vi "CRYPEAQ SpreadCB Sub.vi"(9 "Bs":dbl[](array[numeric]), 10 "Center Frequency":dbl[](array[numeric]), 11 "E":dbl[](array[numeric])) -> (3 "Es":dbl[](array[numeric]))   [LabVIEW 2013]
panel:
  out "Array 2":dbl[](array[numeric])
  out "Array":dbl[](array[numeric])
  out "aUCEe":dbl[](array[numeric])
  out "Ene":dbl[](array[numeric])
  in  "res":dbl=0.25
  out "XY Graph 4":cluster{"Center Frequency":dbl[], "E":dbl[]}[](graph)
  out "size(s) 4":i32
  out "size(s) 3":i32
  out "size(s)":i32
  # "SU Value Range"
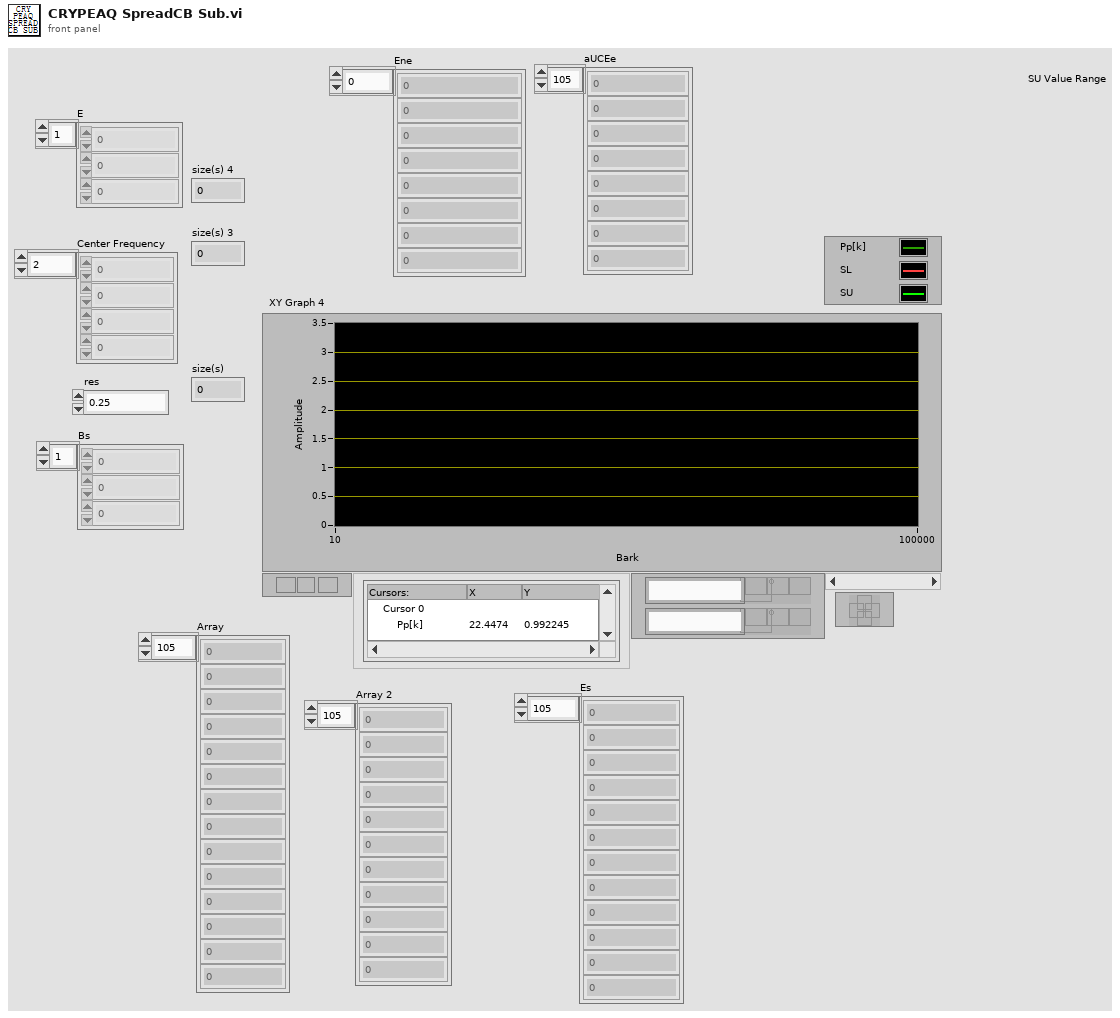
[diagram p1: front panel]
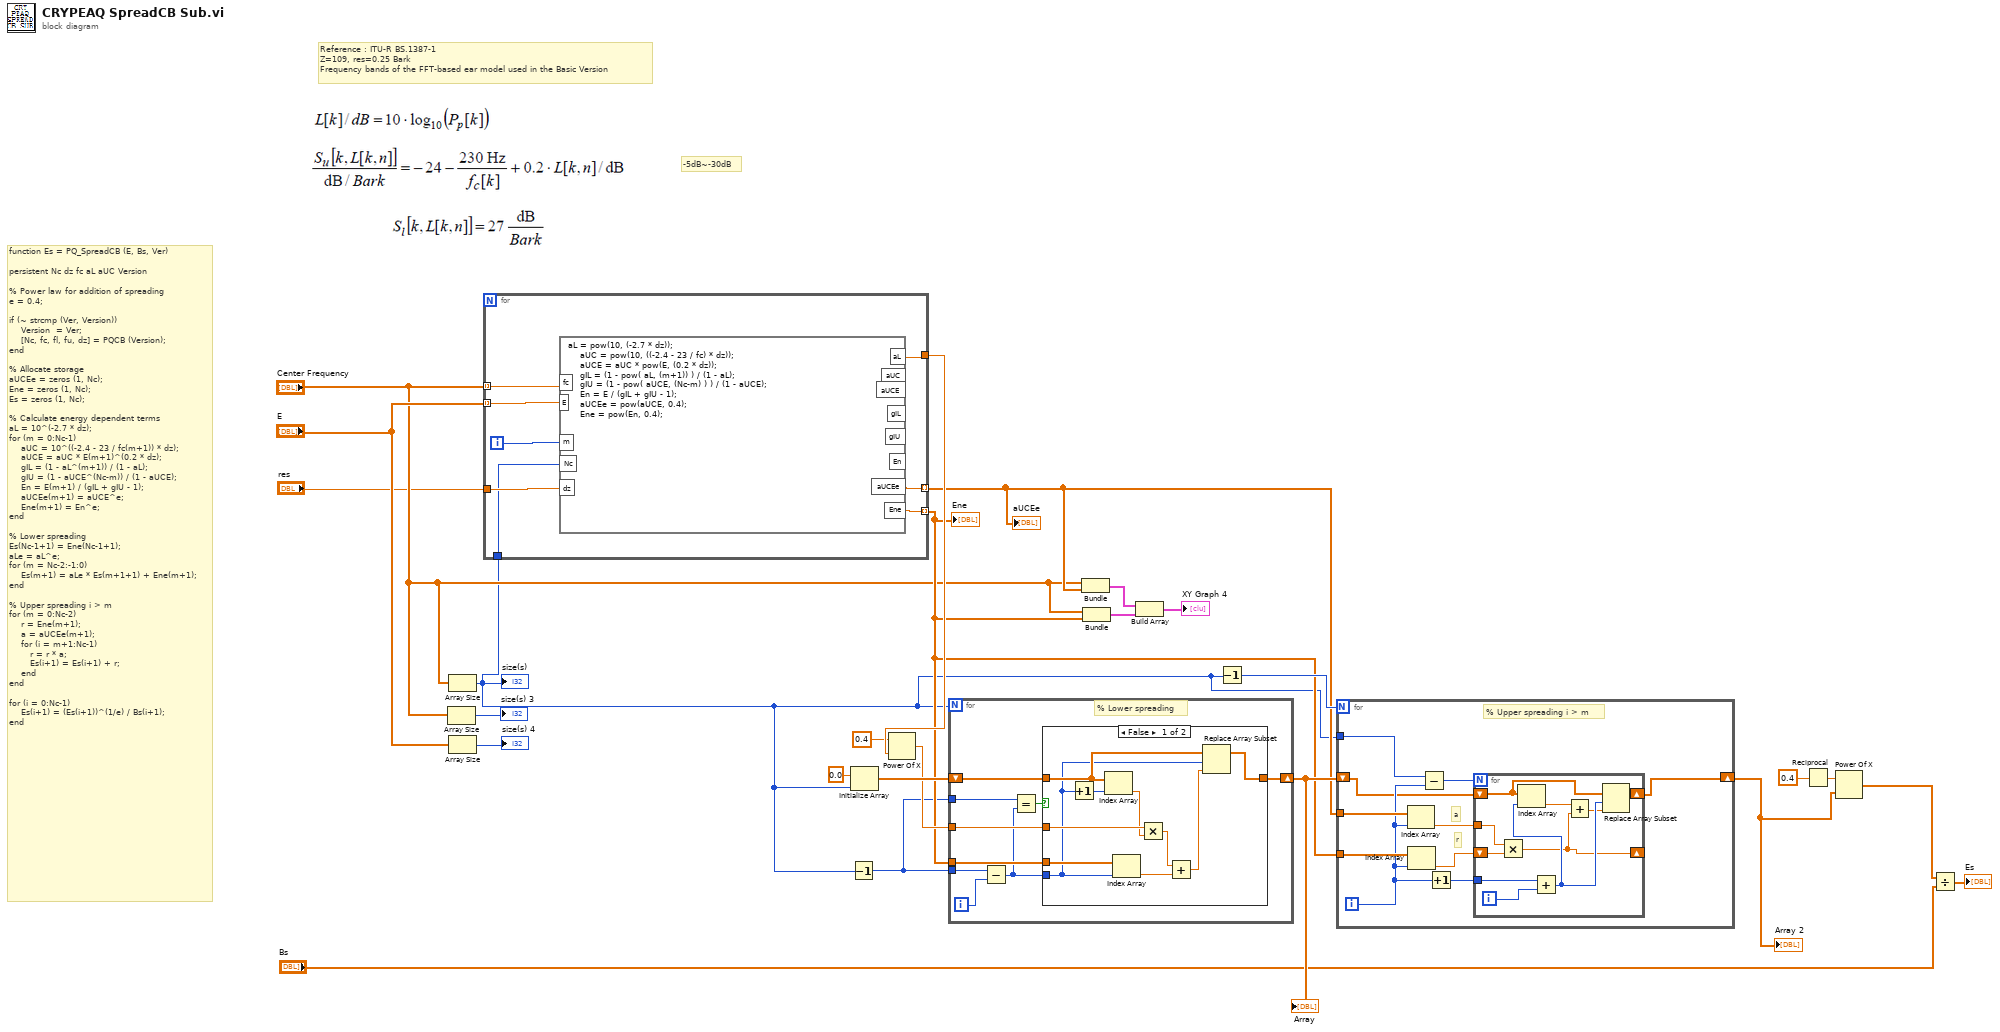
[diagram p0: block diagram]
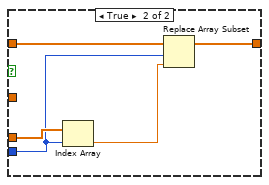
[diagram p2: hidden frame]
diagram:
  # "function Es = PQ_SpreadCB (E, Bs, Ver)\n\npersistent Nc dz fc aL aUC Version\n\n% Power law for addition of spreading\ne = 0.4;\n\nif (~ strcmp (Ver, Version))\n    Version  = Ver;\n    [Nc, fc, fl, fu, dz] = PQCB (Version);\nend\n\n% Allocate storage\naUCEe = zeros (1, Nc);\nEne = zeros (1, Nc);\nEs = zeros (1, Nc);\n\n% Calculate energy dependent terms\naL = 10^(-2.7 * dz);\nfor (m = 0:Nc-1)\n    aUC = 10^((-2.4 - 23 / fc(m+1)) * dz);\n    aUCE = aUC * E(m+1)^(0.2 * dz);\n    gIL = (1 - aL^(m+1)) / (1 - aL);\n    gIU = (1 - aUCE^(Nc-m)) / (1 - aUCE);\n    En = E(m+1) / (gIL + gIU - 1);\n    aUCEe(m+1) = aUCE^e;\n    Ene(m+1) = En^e;\nend\n\n% Lower spreading\nEs(Nc-1+1) = Ene(Nc-1+1);\naLe = aL^e;\nfor (m = Nc-2:-1:0)\n    Es(m+1) = aLe * Es(m+1+1) + Ene(m+1);\nend\n\n% Upper spreading i > m\nfor (m = 0:Nc-2)\n    r = Ene(m+1);\n    a = aUCEe(m+1);\n    for (i = m+1:Nc-1)\n       r = r * a;\n       Es(i+1) = Es(i+1) + r;\n    end\nend\n\nfor (i = 0:Nc-1)\n    Es(i+1) = (Es(i+1))^(1/e) / Bs(i+1);\nend"
  # "Reference : ITU-R BS.1387-1\nZ=109, res=0.25 Bark\nFrequency bands of the FFT-based ear model used in the Basic Version"
  # "-5dB~-30dB"
  n1 = Array Size(array="Center Frequency") -> (size(s)=→"size(s) 3":i32)
  n2 = Array Size(array="Center Frequency") -> (size(s)=w5:i32)
  "size(s)" <- w5
  n3 = Array Size(array="E") -> (size(s)=→"size(s) 4":i32)
  n4 = for {
    tunnel: "E" -> [w32] mode=indexing
    tunnel: "Center Frequency" -> [w33] mode=indexing
    tunnel: "res" -> [w27]
    tunnel: [w30] -> w9 mode=indexing
    tunnel: [w29] -> w15 mode=indexing
    tunnel: [w28] -> w20
    tunnel: w5 -> [w26]
    i -> [w31]
    n5 = formula code="aL = pow(10, (-2.7 * dz));\n    aUC = pow(10, ((-2.4 - 23 / fc) * dz));\n    aUCE = aUC * pow(E, (0.2 * dz));\n    gIL = (1 - pow( aL, (m+1)) ) / (1 - aL);\n    gIU = (1 - pow( aUCE, (Nc-m) ) ) / (1 - aUCE);\n    En = E / (gIL + gIU - 1);\n    aUCEe = pow(aUCE, 0.4);\n    Ene = pow(En, 0.4);"("dz"=w27, "fc"=w33, "E"=w32, "m"=w31, "Nc"=w26) -> ("aL"=w28:dbl, "aUCEe"=w29:dbl, "Ene"=w30:dbl)  [unwired: 5 out]
  }
  "Ene" <- w9
  "aUCEe" <- w15
  n6 = Decrement(x=w5) -> (x-1=w4:i32)
  n7 = Initialize Array(0.0 ("element"), w5) -> (w21:dbl[])
  n8 = Power Of X(1:w20, 2:0.4 ("input variable")) -> (0:w18:dbl)
  n9 = for {
    N: w5 -> [_]
    tunnel: w9 -> [w40]
    shift-right: [w41] -> w17
    shift-left: w21 -> [w42]
    tunnel: w4 -> [w39]
    tunnel: w18 -> [w38]
    tunnel: w4 -> [w37]
    i -> [w36]
    # "% Lower spreading"
    n10 = Subtract(x=w39, y=w36) -> (x-y=w35:i32)
    n11 = Equal?(x=w37, y=w35) -> (x = y?=w34:bool)
    n12 = case shown="False" w34 {
      tunnel: w42 -> [w52 w56]
      tunnel: [w51 w53] -> w41
      tunnel: w40 -> [w50 w57]
      tunnel: w38 -> [w49 _]
      tunnel: w35 -> [w43 w55]
      frame False {
        n13 = Increment(x=w43) -> (x+1=w44:i32)
        n14 = Index Array(array=w52, index=w44) -> (element=w48:dbl)
        n15 = Index Array(array=w50, index=w43) -> (element=w46:dbl)
        n16 = Multiply(x=w49, y=w48) -> (x*y=w47:dbl)
        n17 = Add(x=w47, y=w46) -> (x+y=w45:dbl)
        n18 = Replace Array Subset(array=w52, new element=w45, index=w43) -> (w51:dbl[])
      }
      frame True {
        n19 = Index Array(array=w57, index=w55) -> (element=w54:dbl)
        n20 = Replace Array Subset(array=w56, new element=w54, index=w55) -> (w53:dbl[])
      }
    }
  }
  "Array" <- w17
  n21 = Bundle("Center Frequency"="Center Frequency", w15) -> (w23:cluster{"Center Frequency":dbl[], dbl[]})  [unwired: 1 in]
  n22 = Bundle("Center Frequency"="Center Frequency", w9) -> (w10:cluster{"Center Frequency":dbl[], dbl[]})  [unwired: 1 in]
  n23 = Build Array(w23, w10) -> (→"XY Graph 4":cluster{"Center Frequency":dbl[], dbl[]}[])
  n24 = Decrement(x=w5) -> (x-1=w16:i32)
  n25 = for {
    N: w16 -> [_]
    tunnel: w9 -> [w67]
    shift-right: [w59] -> w3
    shift-left: w17 -> [w60]
    tunnel: w15 -> [w66]
    tunnel: w5 -> [w63]
    i -> [w62]
    # "a"
    # "r"
    # "% Upper spreading i > m"
    n26 = Index Array(array=w66, index=w62) -> (element=w65:dbl)
    n27 = Index Array(array=w67, index=w62) -> (element=w64:dbl)
    n28 = Subtract(x=w63, y=w62) -> (x-y=w61:i32)
    n29 = Increment(x=w62) -> (x+1=w58:i32)
    n30 = for {
      N: w61 -> [_]
      tunnel: w65 -> [w77]
      shift-right: [w69] -> _
      shift-left: w64 -> [w76]
      tunnel: w58 -> [w74]
      shift-right: [w71] -> w59
      shift-left: w60 -> [w72]
      i -> [w75]
      n31 = Multiply(x=w77, y=w76) -> (x*y=w69:dbl)
      n32 = Add(x=w74, y=w75) -> (x+y=w73:i32)
      n33 = Index Array(array=w72, index=w73) -> (element=w70:dbl)
      n34 = Add(x=w70, y=w69) -> (x+y=w68:dbl)
      n35 = Replace Array Subset(array=w72, new element=w68, index=w73) -> (w71:dbl[])
    }
  }
  "Array 2" <- w3
  n36 = Reciprocal(x=0.4) -> (1/x=w2:dbl)
  n37 = Power Of X(1:w3, 2:w2) -> (0:w12:dbl[])
  n38 = Divide(x=w12, y="Bs") -> (x/y=→"Es":dbl[])
